vi "Day 7.1.vi"(11 "input":string[](array[string])) -> (3 "ouptut part 1":u64)   [LabVIEW 2021]
uses:
  af89766b-20e1-4237-9b5b-6081e661f8af.vi
  <vilib>/Comparison/Less/Less Functor/Less Functor.lvclass
panel:
  out "Array":i32[](array[numeric])
  out "appended array":bool[][](array[boolean])
  out "Array 3":T1(array[cluster])
  # "248581821 too high"
  # "32T3K"
  # "KTJJT"
  # "KK677"
  # "T55J5"
  # "QQQJA"
  # "So, the first step is to put the hands in order of strength:\n\n32T3K is the only one pair and the other hands are all a stronger type, so it gets rank 1.\nKK677 and KTJJT are both two pair. Their first cards both have the same label, but the second card of KK677 is stronger (K vs T), so KTJJT gets rank 2 and KK677 gets rank 3.\nT55J5 and QQQJA are both three of a kind. QQQJA has a stronger first card, so it gets rank 5 and T55J5 gets rank 4.\nNow, you can determine the total winnings of this set of hands by adding up the result of multiplying each hand's bid with its rank (765 * 1 + 220 * 2 + 28 * 3 + 684 * 4 + 483 * 5). So the total winnings in this example are 6440."
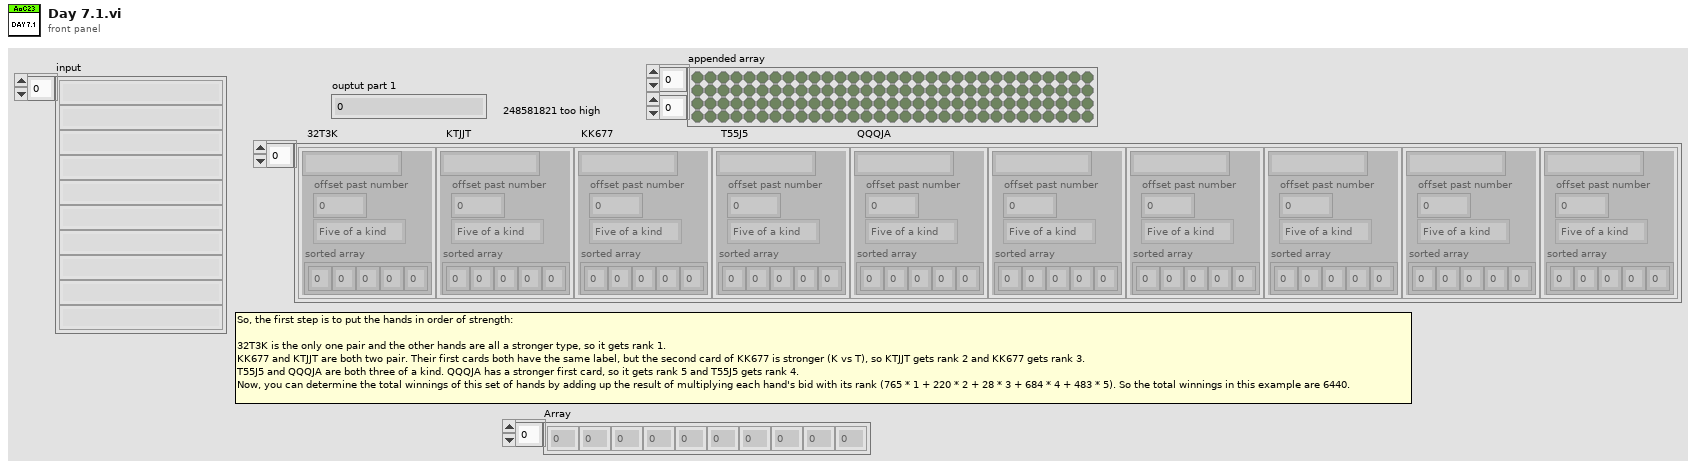
[diagram p1: front panel]
types:
  T1 = cluster{string, "offset past number":u64, enum16{"Five of a kind", "Four of a kind", "Full house", "Three of a kind", "Two pair", "One pair", "High card"}, "sorted array":u8[]}[]
  T2 = cluster{"Hand":string, "Value":u64, "Type":enum16{"Five of a kind", "Four of a kind", "Full house", "Three of a kind", "Two pair", "One pair", "High card"}, "Array":u8[]}[]
  T3 = cluster{"Hand":string, "Value":u64, "Type":enum16{"Five of a kind", "Four of a kind", "Full house", "Three of a kind", "Two pair", "One pair", "High card"}, "Array":u8[]}
  T4 = enum16{"Five of a kind", "Four of a kind", "Full house", "Three of a kind", "Two pair", "One pair", "High card"}
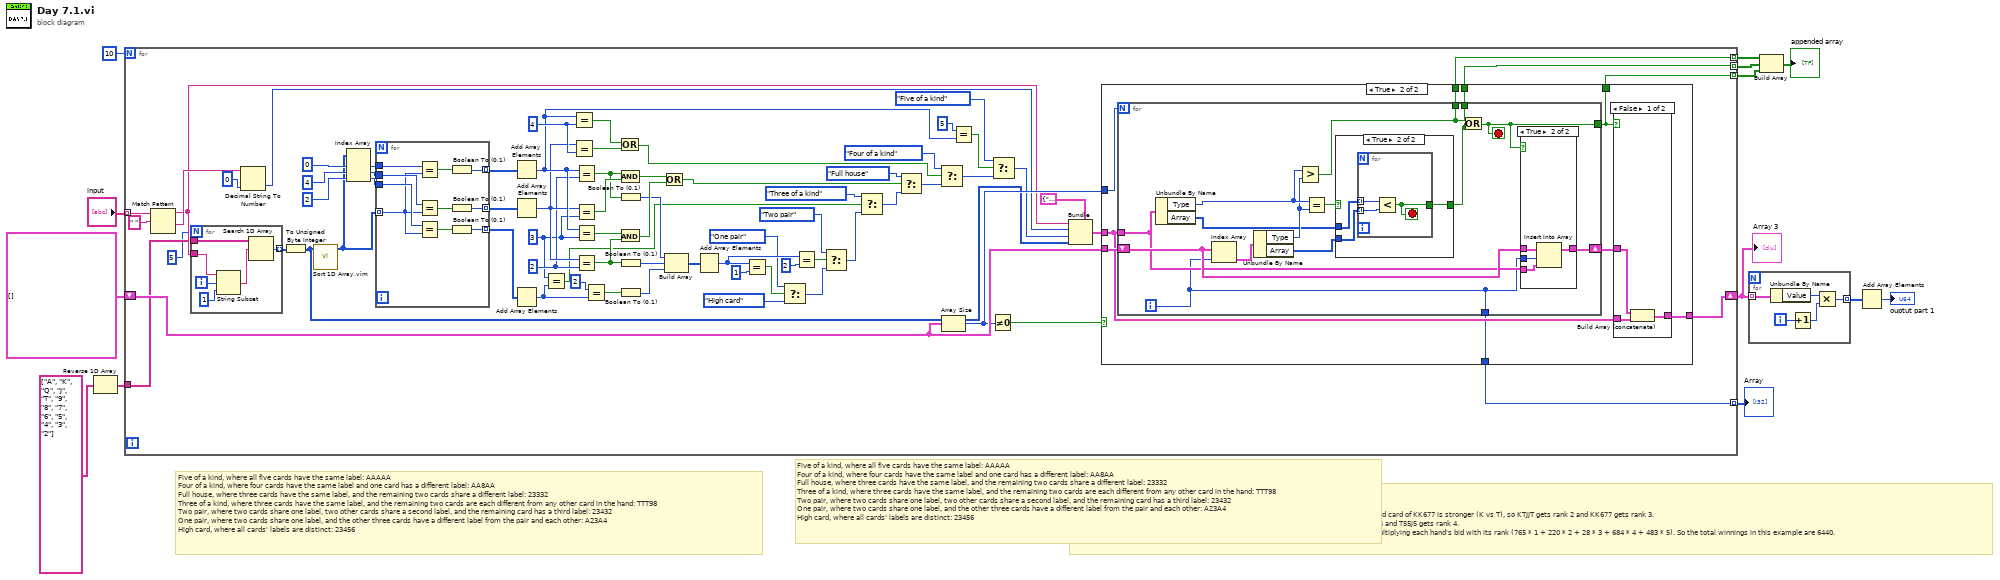
[diagram p0: block diagram]
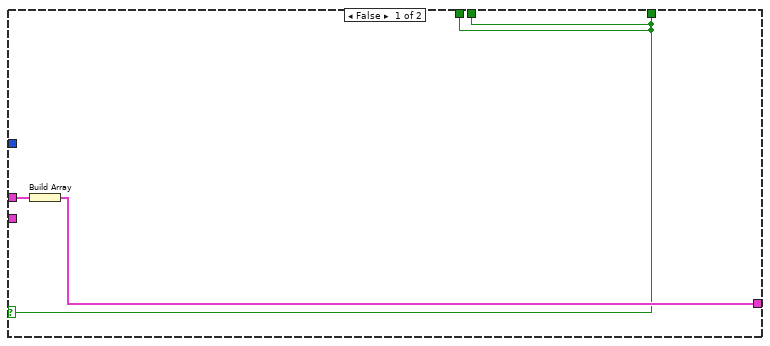
[diagram p2: hidden frame]
diagram:
  # "Five of a kind, where all five cards have the same label: AAAAA\nFour of a kind, where four cards have the same label and one card has a different label: AA8AA\nFull house, where three cards have the same label, and the remaining two cards share a different label: 23332\nThree of a kind, where three cards have the same label, and the remaining two cards are each different from any other card in the hand: TTT98\nTwo pair, where two cards share one label, two other cards share a second label, and the remaining card has a third label: 23432\nOne pair, where two cards share one label, and the other three cards have a different label from the pair and each other: A23A4\nHigh card, where all cards' labels are distinct: 23456"
  # "So, the first step is to put the hands in order of strength:\n\n32T3K is the only one pair and the other hands are all a stronger type, so it gets rank 1.\nKK677 and KTJJT are both two pair. Their first cards both have the same label, but the second card of KK677 is stronger (K vs T), so KTJJT gets rank 2 and KK677 gets rank 3.\nT55J5 and QQQJA are both three of a kind. QQQJA has a stronger first card, so it gets rank 5 and T55J5 gets rank 4.\nNow, you can determine the total winnings of this set of hands by adding up the result of multiplying each hand's bid with its rank (765 * 1 + 220 * 2 + 28 * 3 + 684 * 4 + 483 * 5). So the total winnings in this example are 6440."
  # "Five of a kind, where all five cards have the same label: AAAAA\nFour of a kind, where four cards have the same label and one card has a different label: AA8AA\nFull house, where three cards have the same label, and the remaining two cards share a different label: 23332\nThree of a kind, where three cards have the same label, and the remaining two cards are each different from any other card in the hand: TTT98\nTwo pair, where two cards share one label, two other cards share a second label, and the remaining card has a third label: 23432\nOne pair, where two cards share one label, and the other three cards have a different label from the pair and each other: A23A4\nHigh card, where all cards' labels are distinct: 23456"
  n1 = Reverse 1D Array(array=string[] ["A", "K", "Q", "J", "T", "9", "8", "7", "6", "5", "4", "3", "2"]) -> (reversed array=w7:string[])
  n2 = for {
    N: 10 -> [_]
    tunnel: "input" -> [w86] mode=indexing
    shift-right: [w33] -> w9
    shift-left: T2 [] -> [w32]
    tunnel: w7 -> [w24]
    tunnel: [w17] -> w3 mode=indexing
    tunnel: [w16] -> w5 mode=indexing
    tunnel: [w15] -> w4 mode=indexing
    tunnel: [w14] -> w1 mode=indexing
    w20 = i16 3 ("y")
    w61 = i16 2 ("y")
    w74 = i16 4 ("y")
    n3 = Match Pattern(string=w86, regular expression=" ") -> (before substring=w25:string, after substring=w84:string)  [unwired: 1 in, 2 out]
    n4 = for {
      N: 5 -> [_]
      tunnel: w25 -> [w92]
      tunnel: w24 -> [w89]
      tunnel: [w87] -> w22 mode=indexing
      i -> [w91]
      n5 = String Subset(string=w92, offset (0)=w91, length (rest)=1 ("length (rest)")) -> (substring=w88:string)
      n6 = Search 1D Array(1D array=w89, element=w88) -> (index of element=w87:i32)  [unwired: 1 in]
    }
    n7 = Decimal String To Number(string=w84, default (0L)=u64 0 ("default (0 I32)")) -> (number=w28:u64)  [unwired: 1 in, 1 out]
    n8 = To Unsigned Byte Integer(number=w22) -> (unsigned 8bit integer=w18:u8[])
    n9 = call "Sort 1D Array.vim"("unsorted array"=w18) -> ("sorted array"=w34:u8[])  [unwired: 10 in]
    n10 = Index Array(array=w34, index #1=0 ("index"), index #2=4 ("index"), index #3=2 ("index")) -> (element #1=w83:u8, element #2=w80:u8, element #3=w55:u8)
    n11 = for {
      tunnel: w34 -> [w136] mode=indexing
      tunnel: w83 -> [w143]
      tunnel: w80 -> [w141]
      tunnel: [w139] -> w79 mode=indexing
      tunnel: [w138] -> w78 mode=indexing
      tunnel: w55 -> [w137]
      tunnel: [w134] -> w54 mode=indexing
      n12 = Equal?(x=w143, y=w136) -> (x = y?=w142:bool)
      n13 = Equal?(x=w141, y=w136) -> (x = y?=w140:bool)
      n14 = Equal?(x=w137, y=w136) -> (x = y?=w135:bool)
      n15 = Boolean To (0,1)(Boolean=w142) -> (0, 1=w139:i16)
      n16 = Boolean To (0,1)(Boolean=w140) -> (0, 1=w138:i16)
      n17 = Boolean To (0,1)(Boolean=w135) -> (0, 1=w134:i16)
    }
    n18 = Add Array Elements(numeric array=w79) -> (sum=w63:i16)
    n19 = Add Array Elements(numeric array=w78) -> (sum=w62:i16)
    n20 = Add Array Elements(numeric array=w54) -> (sum=w21:i16)
    n21 = Equal?(x=w20, y=w21) -> (x = y?=w19:bool)
    n22 = Equal?(x=w63, y=w74) -> (x = y?=w73:bool)
    n23 = Equal?(x=w62, y=w74) -> (x = y?=w72:bool)
    n24 = Equal?(x=w63, y=w61) -> (x = y?=w51:bool)
    n25 = Equal?(x=w62, y=w20) -> (x = y?=w58:bool)
    n26 = Equal?(x=w63, y=w20) -> (x = y?=w57:bool)
    n27 = Equal?(x=w62, y=w61) -> (x = y?=w50:bool)
    n28 = Equal?(x=i16 2 ("y"), y=w21) -> (x = y?=w52:bool)
    n29 = Or(x=w73, y=w72) -> (x .or. y?=w71:bool)
    n30 = And(x=w51, y=w58) -> (x .and. y?=w66:bool)
    n31 = Boolean To (0,1)(Boolean=w51) -> (0, 1=w49:i16)
    n32 = And(x=w57, y=w50) -> (x .and. y?=w65:bool)
    n33 = Boolean To (0,1)(Boolean=w50) -> (0, 1=w48:i16)
    n34 = Boolean To (0,1)(Boolean=w52) -> (0, 1=w47:i16)
    n35 = Or(x=w66, y=w65) -> (x .or. y?=w64:bool)
    n36 = Build Array(w49, w48, w47) -> (w46:i16[])
    n37 = Add Array Elements(numeric array=w46) -> (sum=w45:i16)
    n38 = Equal?(x=w45, y=i16 1) -> (x = y?=w41:bool)
    n39 = Select(t=T4."One pair", s=w41, f=T4."High card") -> (s? t:f=w36:T4)
    n40 = Equal?(x=w45, y=i16 2) -> (x = y?=w40:bool)
    n41 = Select(t=T4."Two pair", s=w40, f=w36) -> (s? t:f=w39:T4)
    n42 = Select(t=T4."Three of a kind", s=w19, f=w39) -> (s? t:f=w60:T4)
    n43 = Select(t=T4."Full house", s=w64, f=w60) -> (s? t:f=w67:T4)
    n44 = Select(t=T4."Four of a kind", s=w71, f=w67) -> (s? t:f=w69:T4)
    n45 = Array Size(array=w32) -> (size(s)=w31:i32)
    n46 = Equal?(x=i16 5 ("y"), y=w63) -> (x = y?=w76:bool)
    n47 = Not Equal To 0?(x=w31) -> (x != 0?=w30:bool)
    n48 = Select(t=T4."Five of a kind", s=w76, f=w69) -> (s? t:f=w27:T4)
    n49 = Bundle(cluster=T3 {"Hand"="", "Value"=0, "Type"=enum."Five of a kind", "Array"=[]} ("output cluster"), "Hand"=w25, "Value"=w28, "Type"=w27, "Array"=w18) -> (w26:T3)
    n50 = case shown="True" w30 {
      selector: w30 -> [w93 _]
      tunnel: [w94 w101] -> w33
      tunnel: w32 -> [_ w104]
      tunnel: w31 -> [_ w103]
      tunnel: w26 -> [w95 w100]
      tunnel: [w93 w99] -> w17
      tunnel: [w93 w98] -> w16
      tunnel: [w93 w97] -> w15
      tunnel: [_ w96] -> w14
      frame False {
        n51 = Build Array(w95) -> (w94:T2)
      }
      frame True {
        n52 = for {
          N: w103 -> [_]
          shift-right: [w119] -> w102
          shift-left: w104 -> [w120]
          tunnel: w100 -> [w118]
          tunnel: [w112] -> w99
          tunnel: [w111] -> w98
          tunnel: [w110] -> w97
          tunnel: [w109] -> w96
          i -> [w109]
          stop <- w112 stop-if-true
          n53 = Unbundle By Name(w118) -> ("Type"=w117:T4, "Array"=w113:u8[])
          n54 = Index Array(array=w120, index=w109) -> (element=w121:T3)
          n55 = Unbundle By Name(w121) -> ("Type"=w116:T4, "Array"=w114:u8[])
          n56 = Greater?(x=w117, y=w116) -> (0:w111:bool)
          n57 = Equal?(x=w117, y=w116) -> (x = y?=w115:bool)
          n58 = case shown="True" w115 {
            selector: w115 -> [w122 _]
            tunnel: w114 -> [_ w124]
            tunnel: w113 -> [_ w125]
            tunnel: [w122 w123] -> w110
            frame False {
            }
            frame True {
              n59 = for {
                tunnel: w125 -> [w128] mode=indexing
                tunnel: w124 -> [w127] mode=indexing
                tunnel: [w126] -> w123
                stop <- w126 stop-if-true
                n60 = Less?(x=w128, y=w127) -> (x < y?=w126:bool)
              }
            }
          }
          n61 = Or(x=w111, y=w110) -> (x .or. y?=w112:bool)
          n62 = case shown="True" w112 {
            tunnel: w120 -> [w129 w133]
            tunnel: [w129 w132] -> w119
            tunnel: w118 -> [_ w131]
            tunnel: w109 -> [_ w130]
            frame False {
            }
            frame True {
              n63 = Insert Into Array(array=w133, index=w130, new element=w131) -> (w132:T2)
            }
          }
        }
        n64 = case shown="False" w99 {
          tunnel: w102 -> [w107 w108]
          tunnel: [w106 w108] -> w101
          tunnel: w100 -> [w105 _]
          frame False {
            n65 = Build Array (concatenate)(w107, w105) -> (w106:T2)
          }
          frame True {
          }
        }
      }
    }
  }
  "Array 3" <- w9
  "Array" <- w1
  n66 = for {
    tunnel: w9 -> [w148] mode=indexing
    tunnel: [w144] -> w10 mode=indexing
    i -> [w146]
    n67 = Unbundle By Name(w148) -> ("Value"=w147:u64)
    n68 = Increment(x=w146) -> (x+1=w145:i32)
    n69 = Multiply(x=w147, y=w145) -> (x*y=w144:u64)
  }
  n70 = Build Array(w5, w4, w3) -> (→"appended array":bool[][])
  n71 = Add Array Elements(numeric array=w10) -> (sum=→"ouptut part 1":u64)
